vi "Stop Core.vi"(10 "final error code":i32, 11 "HIJ Vision Camera App w Timer in":refnum<class "HIJ Vision Camera App w Timer.lvclass">) -> (3 "HIJ Vision Camera App w Timer out":refnum<class "HIJ Vision Camera App w Timer.lvclass">)   [LabVIEW 2014, in "HIJ Vision Camera App w Timer.lvlib" / "HIJ Vision Camera App w Timer.lvclass"]
doc: "(<B>Filename</B>: Actor Framework.lvlib:Actor.lvclass:Stop Core.vi)\n\nDefines what the actor does before it stops. Use the <B>final error code</B> input to determine whether the actor shut down in response to an error.\n\nBy default, this method does nothing. A descendant class may override it to define behavior, such as shutting down any processes the actor initiated in its override of the Actor Core method."
uses:
  HIJ Vision Camera App w Timer.lvclass
  <vilib>/ActorFramework/Time-Delayed Send Message/Time-Delay Override Options.ctl
  HIJ Vision Camera App w Timer.lvclass/HIJ Vision Camera App w Timer.ctl
  Applications/HIJ Vision Camera App/HIJ Vision Camera App/HIJ Vision Camera App.lvclass
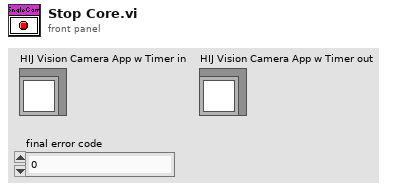
[diagram p1: front panel]
types:
  T1 = typedef "Time-Delay Override Options.ctl" = enum16{"Send next copy now", "Skip next scheduled copy", "Send next copy now and stop all further copies", "Stop all further copies"}
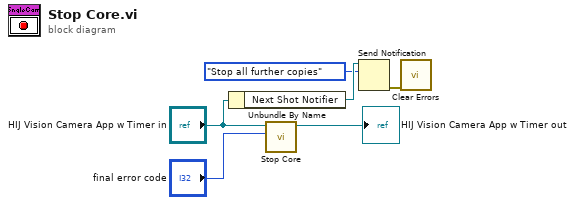
[diagram p0: block diagram]
diagram:
  n1 = Unbundle By Name("HIJ Vision Camera App w Timer in") -> ("Next Shot Notifier"=w3:refnum<notifier>)
  n2 = call-parent "Stop Core.vi"("final error code"="final error code", "ViewableActor in"="HIJ Vision Camera App w Timer in") -> ("ViewableActor out"=→"HIJ Vision Camera App w Timer out":refnum<class "HIJ Vision Camera App w Timer.lvclass">)  [unwired: 9 in]
  n3 = Send Notification(notification=Time-Delay_Override_Options."Stop all further copies", notifier=w3) -> (error out=w1:errorcluster)  [unwired: 1 in, 1 out]
  n4 = call <vilib>:"Clear Errors.vi"("error in (no error)"=w1) -> ()  [unwired: 5 in, 2 out]
